vi "ExSubCreateDisplay.vi"(2 "error in (no error)":errorcluster, 3 "File and Display Name":string, 4 "Pulser Handle":u32, 5 "Camera Handle":u32) -> (0 "error out":errorcluster, 1 "Handles Out":T1)   [LabVIEW 2010]
panel:
  # "ExSubCreateDisplay:\nThis is a SubVI that creates display and image \nobjects and returns the handles bundled in a \ncluster that includes a pulser and camera handle"
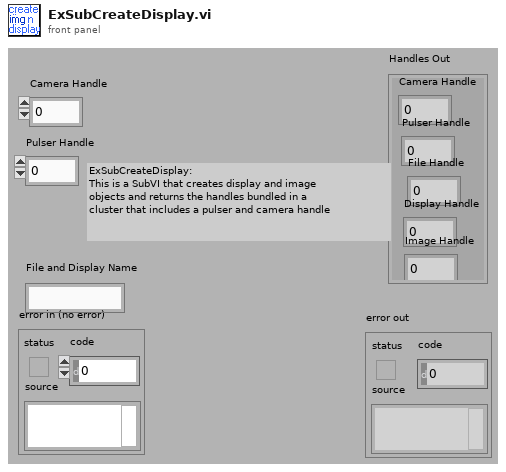
[diagram p1: front panel]
types:
  T1 = cluster{"Camera Handle":u32, "Pulser Handle":u32, "File Handle":u32, "Display Handle":u32, "Image Handle":u32}
  T2 = cluster{"Camera Handle":u32, "Pulser Handle":u32, i32, "Display Handle":u32, "Image Handle":u32}
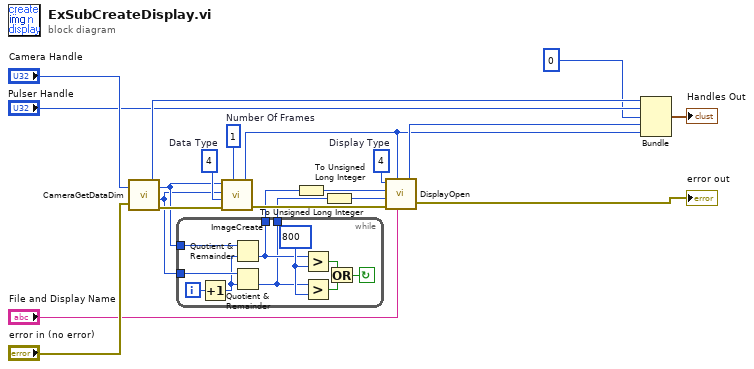
[diagram p0: block diagram]
diagram:
  w10 = u32 1  # Number Of Frames
  w11 = u32 4  # Display Type
  w12 = u32 4  # Data Type
  n1 = call <userlib>:"CameraGetDataDim.vi"("Camera Handle"="Camera Handle", "error in"="error in (no error)") -> ("Camera Handle"=w17:u32, "Xdim"=w9:u32, "Ydim"=w8:u32, "error out"=w21:errorcluster)
  n2 = while {
    tunnel: w9 -> [w30]
    tunnel: w8 -> [w29]
    tunnel: [w24] -> w7
    tunnel: [w23] -> w6
    i -> [w28]
    stop <- w25 continue-if-true
    w31 = 800
    n3 = Increment(x=w28) -> (x+1=w22:i32)
    n4 = Quotient & Remainder(x=w30, y=w22) -> (floor(x/y)=w24:u32)  [unwired: 1 out]
    n5 = Quotient & Remainder(x=w29, y=w22) -> (floor(x/y)=w23:u32)  [unwired: 1 out]
    n6 = Greater?(x=w24, y=w31) -> (0:w27:bool)
    n7 = Greater?(x=w23, y=w31) -> (0:w26:bool)
    n8 = Or(x=w27, y=w26) -> (x .or. y?=w25:bool)
  }
  n9 = call <userlib>:"ImageCreate.vi"("X dimension"=w9, "Y dimension"=w8, "Data Type"=w12, "error in"=w21, "Number Of Frames"=w10) -> ("Image Handle"=w14:u32, "error out"=w20:errorcluster)
  n10 = To Unsigned Long Integer(number=w7) -> (unsigned 32bit integer=w5:u32)
  n11 = To Unsigned Long Integer(number=w6) -> (unsigned 32bit integer=w4:u32)
  n12 = call <userlib>:"DisplayOpen.vi"("Display Title"="File and Display Name", "Image Handle"=w14, "error in"=w20, "Display Height"=w4, "Display Width"=w5, "Display Type"=w11) -> ("error out"=→"error out":errorcluster, "Display Handle"=w15:u32)
  n13 = Bundle("Camera Handle"=w17, "Pulser Handle"="Pulser Handle", 0, "Display Handle"=w15, "Image Handle"=w14) -> (→"Handles Out":T2)  [unwired: 1 in]
